vi "SVT UFF58 Read Record 8.vi"(0 "function refnum":refnum<k20>, 11 "error in (no error)":errorcluster) -> (4 "dup function refnum":refnum<k20>, 6 "abscissa data characteristics":T1 {"specific data type" items=["unknown"=0, "general"=1, "stress"=2, "strain"=3, "temperature"=5, "heat flux"=6, "displacement"=8, "reaction force"=9, "velocity"=11, "acceleration"=12, "excitation force"=13, "pressure"=15, "mass"=16, "time"=17, "frequency"=18, "rpm"=19, "order"=20, "sound pressure"=21, "sound intensity"=22, "sound power"=23]}, 15 "error out":errorcluster)   [LabVIEW 2017, in "SoundVib_UFF58.lvlib"]
doc: "Reads the values of all the fields in record 8 of a UFF58 (universal file format) file. Record 8 contains the abscissa data characteristics."
uses:
  <vilib>/addons/Sound and Vibration/svt_UFF58/SoundVib_UFF58.lvlib
  <vilib>/addons/Sound and Vibration/svt_UFF58/subVIs/sv_UFF58 Axis Characteristics.ctl
  <vilib>/addons/Sound and Vibration/svt_UFF58/subVIs/sv_UFF58 Specific Datatype.ctl
  <vilib>/Platform/storage/Storage.llb/Get Property (String).vi
  <vilib>/Platform/storage/Storage.llb/Get Property (I32).vi
  <vilib>/Platform/storage/Storage.llb/Get Property (Storage Refnums).vi
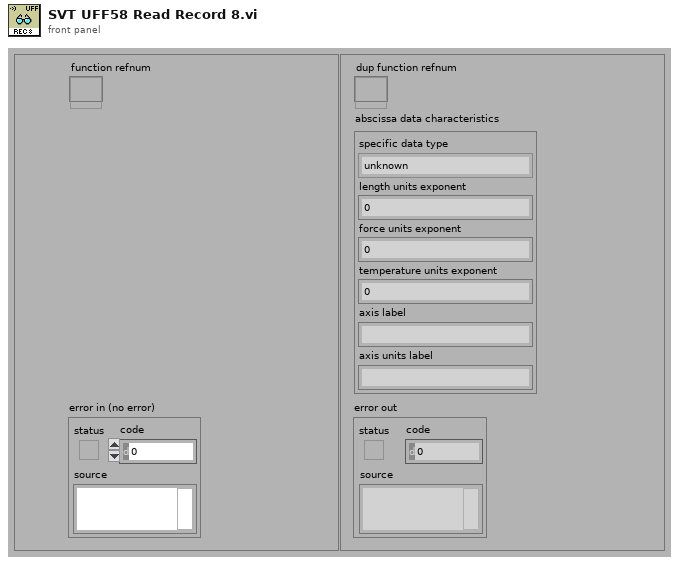
[diagram p1: front panel]
types:
  T1 = typedef "SoundVib_UFF58.lvlib/sv_UFF58 Axis Characteristics.ctl" = cluster{"specific data type":T2, "length units exponent":i32, "force units exponent":i32, "temperature units exponent":i32, "axis label":string, "axis units label":string}
  T2 = typedef "SoundVib_UFF58.lvlib/sv_UFF58 Specific Datatype.ctl" = u16
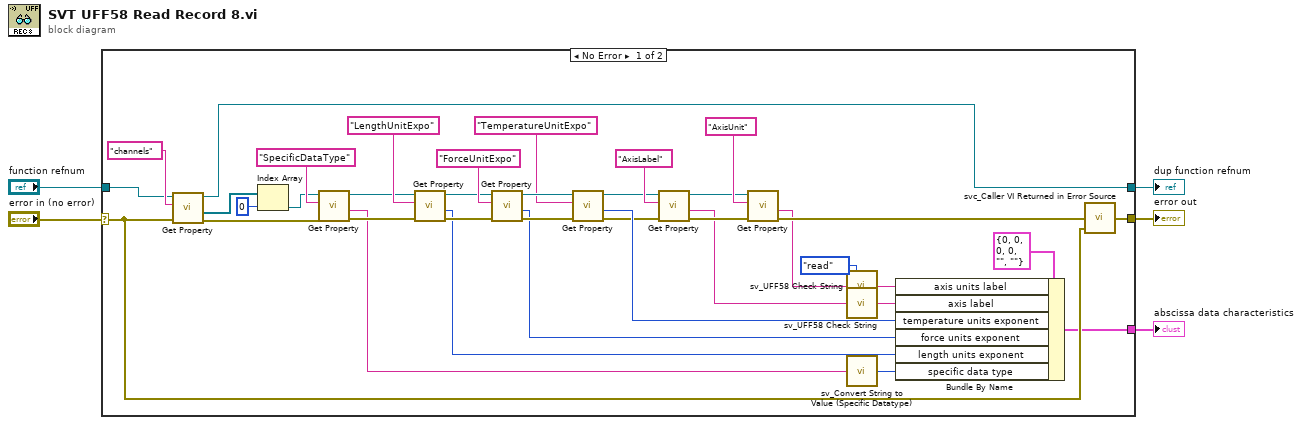
[diagram p0: block diagram]
diagram:
  n1 = case shown="No Error" "error in (no error)" {
    selector: "error in (no error)" -> [w17 w44]
    tunnel: "function refnum" -> [w39 w45]
    tunnel: [w36 w45] -> w2
    tunnel: [w18 w44] -> w5
    tunnel: [w16 _] -> w4
    frame No Error {
      w13 = enum16{"read", "write"}."read" ("operation")
      n2 = call-poly <vilib>:"Get Property.vi"("error in (no error)"=w17, "Property name"="channels", "storage refnum"=w39) -> ("error out"=w38:errorcluster, "Value"=w40:refnum<k20>[], "storage refnum out"=w36:refnum<k20>)  [unwired: 6 in]
      n3 = Index Array(array=w40, index=0) -> (element=w37:refnum<k20>)
      n4 = call-poly <vilib>:"Get Property.vi"("error in (no error)"=w38, "Property name"="SpecificDataType", "storage refnum"=w37) -> ("error out"=w33:errorcluster, "Value"=w12:string, "storage refnum out"=w32:refnum<k20>)  [unwired: 6 in]
      n5 = call-poly <vilib>:"Get Property.vi"("error in (no error)"=w33, "Property name"="LengthUnitExpo", "storage refnum"=w32) -> ("error out"=w29:errorcluster, "Value"=w8:i32, "storage refnum out"=w30:refnum<k20>)  [unwired: 6 in]
      n6 = call-poly <vilib>:"Get Property.vi"("error in (no error)"=w29, "Property name"="ForceUnitExpo", "storage refnum"=w30) -> ("error out"=w27:errorcluster, "Value"=w6:i32, "storage refnum out"=w28:refnum<k20>)  [unwired: 6 in]
      n7 = call-poly <vilib>:"Get Property.vi"("error in (no error)"=w27, "Property name"="TemperatureUnitExpo", "storage refnum"=w28) -> ("error out"=w22:errorcluster, "Value"=w25:i32, "storage refnum out"=w23:refnum<k20>)  [unwired: 6 in]
      n8 = call-poly <vilib>:"Get Property.vi"("error in (no error)"=w22, "Property name"="AxisLabel", "storage refnum"=w23) -> ("error out"=w20:errorcluster, "Value"=w15:string, "storage refnum out"=w21:refnum<k20>)  [unwired: 6 in]
      n9 = call-poly <vilib>:"Get Property.vi"("error in (no error)"=w20, "Property name"="AxisUnit", "storage refnum"=w21) -> ("error out"=w19:errorcluster, "Value"=w14:string)  [unwired: 6 in, 1 out]
      n10 = call <vilib>:"sv_UFF58 Check String.vi"("operation"=w13, "field value"=w14) -> ("output string"=w9:string)  [unwired: 12 in, 1 out]
      n11 = call <vilib>:"sv_UFF58 Check String.vi"("operation"=w13, "field value"=w15) -> ("output string"=w7:string)  [unwired: 12 in, 1 out]
      n12 = call <vilib>:"sv_Convert String to Value (Specific Datatype).vi"("specific data type string"=w12) -> ("specific data type value"=w10:T2)  [unwired: 14 in]
      n13 = Bundle By Name(cluster=T1 {"specific data type"=0, "length units exponent"=0, "force units exponent"=0, "temperature units exponent"=0, "axis label"="", "axis units label"=""} ("abscissa data characteristics"), "axis units label"=w9, "axis label"=w7, "temperature units exponent"=w25, "force units exponent"=w6, "length units exponent"=w8, "specific data type"=w10) -> (w16:T1)
      n14 = call <vilib>:"svc_Caller VI Returned in Error Source.vi"("warning input to caller"=w17, "error in (no error)"=w19) -> ("error out"=w18:errorcluster)  [unwired: 3 in]
    }
    frame Error {
    }
  }
  "error out" <- w5
  "abscissa data characteristics" <- w4
  "dup function refnum" <- w2
